vi "Mesh Page.vi"() -> ()   [LabVIEW 2017, in "3D Mesh.lvclass"]
uses:
  <vilib>/Math Plots/3D Math Plots/3D Mesh/3D Mesh/3D Mesh.lvclass
  <vilib>/Math Plots/3D Math Plots/3D Mesh/3D Mesh/Typedef/3D Mesh Propery Array.ctl
  <vilib>/Math Plots/3D Math Plots/3D Mesh/3D Mesh/Typedef/3D Mesh Property.ctl
  <vilib>/Math Plots/3D Math Plots/3D Plot/3D Plot/Typedef/Line Type.ctl
  <vilib>/Math Plots/3D Math Plots/3D Plot/3D Plot/Typedef/Color Ramp Cluster.ctl
  <vilib>/Math Plots/3D Math Plots/3D Plot/3D Plot/Typedef/Dialog State.ctl
  <vilib>/Math Plots/3D Math Plots/3D Plot/3D Plot/Typedef/Temp Scene State.ctl
  <vilib>/Math Plots/3D Math Plots/3D Plot/3D Plot/Typedef/Temp Scene Property Action.ctl
  <vilib>/Math Plots/3D Math Plots/3D Plot/3D Plot/3D Plot.lvclass
panel:
  in  "Mesh Mode":u16(ring)=2 caption="Mesh mode" items=["Lines", "Hidden Lines", "With Zero Plane"]
  in  "Line Style":u16(ring) caption="Line style"
  in  "Antialiasing":bool
  in  "Line Width":sgl=0.001 caption="Line width" min=0.001 step=1
  in  "Fill Color":u32(colorbox) caption="Fill color"
  out "Mesh Property Out":T1
  in  "Mesh Property In":T1
  out "Color Ramp":dbl[][](graph)
  in  "Color Map Style":u16(ring) caption="Color map style" items=["None ", "Shaded", "Color spectrum", "Grey scale", "Custom"]
  in  "YZ Plane Projection":bool caption="YZ plane projection"
  in  "XZ Plane Projection":bool caption="XZ plane projection"
  in  "XY Plane Projection":bool caption="XY plane projection"
  in  "Coordinate System":u16(ring) caption="Coordinate system" items=["Cartesian", "Cylindrical", "Spherical"]
  in  "Plot Opacity":sgl(slide) caption="Plot opacity(%)" min=0 max=100 scale=0.0..100.0
  in  "Plot List":i32(listbox)
  in  "Ramp Edit":bool caption="Ramp edit"
  in  "Move Down":bool
  in  "Move Up":bool
  in  "Delete":bool
  in  "New":bool
  in  "Event Registration":refnum<event-registration>
  # "Mesh"
  # "General"
  # "Projection"
  # "Color Ramp"
  # "Mesh"
  # "Surface"
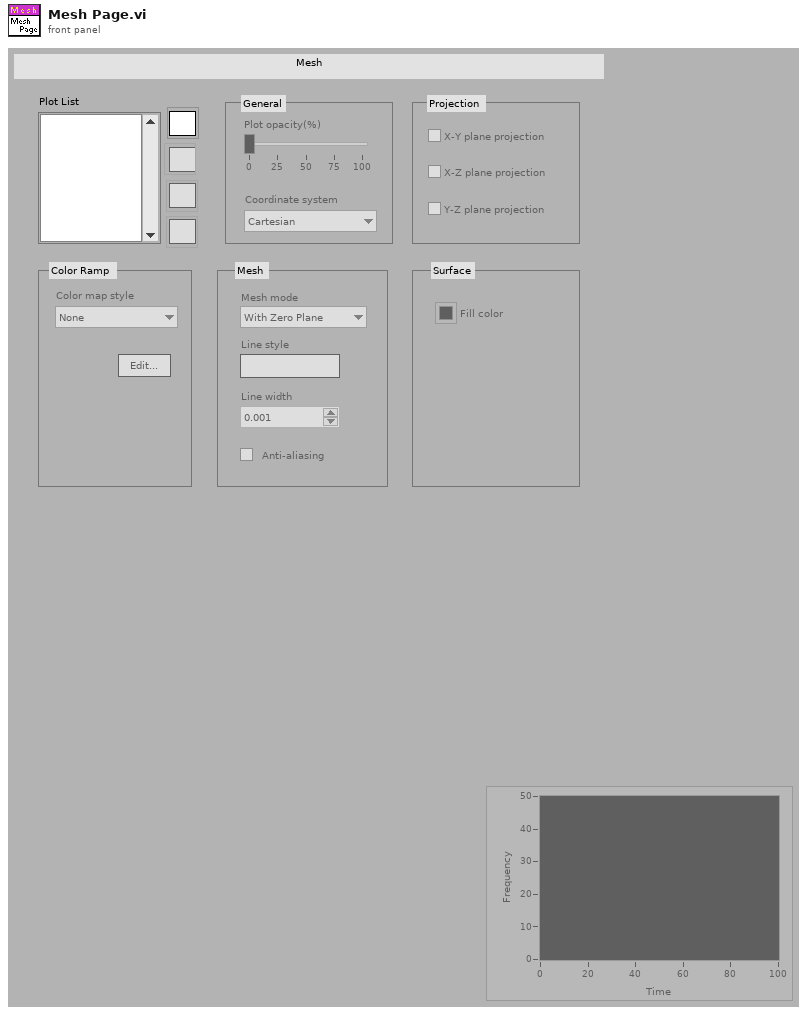
[diagram p1: front panel]
types:
  T1 = typedef "3D Mesh.lvclass/3D Mesh Propery Array.ctl" = T2[]
  T2 = typedef "3D Mesh.lvclass/3D Mesh Property.ctl" = cluster{"General Property":cluster{"Plot Name":string, "Coordinate System":enum16{"Cartesian", "Cylindrical", "Spherical"}, "Opacity":sgl}, "Projection Property":cluster{"Draw XY":bool, "Draw YZ":bool, "Draw XZ":bool}, "Plot Property":cluster{"Surface Color":u32, "Line Style":T3, "Line Width":sgl, "Color Ramp Cluster":T4, "Antialiasing":bool}, "Mesh Property":cluster{"Mesh Mode":enum16{"Lines", "Hidden Lines", "With Zero Plane"}}}
  T3 = typedef "3D Plot.lvclass/Line Type.ctl" = enum16{"None", "Solid", "Dash", "Dot", "Dash Dot"}
  T4 = typedef "3D Plot.lvclass/Color Ramp Cluster.ctl" = cluster{"Color Ramp Style":enum16{"None", "Shaded", "Color spectrum", "Grey scale", "Custom"}, "Color Ramp Array":u32[], "Color Ramp Index":i32[], "Interpolate?":bool, "Logarithm?":bool}
  T5 = typedef "3D Plot.lvclass/Dialog State.ctl" = enum16{"Initialize", "Read Porperty", "Write Property", "Idle", "Exit"}
  T6 = typedef "3D Plot.lvclass/Temp Scene State.ctl" = enum16{"Create", "Update Scene", "Get Plot Representation", "Destory"}
  T7 = typedef "3D Plot.lvclass/Temp Scene Property Action.ctl" = enum16{"Graph Property", "Light Property", "Axis Property", "Value Pair Property", "Format Property", "Cursor Property", "Plot Specific Property"}
  T8 = typedef "3D Plot.lvclass/Multiplot Representation.ctl" = cluster{"Plot Represention Array":T9[], "Max Range":T10}
  T9 = typedef "3D Plot.lvclass/Plot Representation.ctl" = cluster{"Plot ID":i32, "Plot Range":T10, "Mesh Data":T11, "Dimension":cluster{"X Dimension":i32, "Y Dimension":i32}, "Ramp Range":T10}
  T10 = typedef "3D Plot.lvclass/Range Clusters.ctl" = cluster{"X Range":cluster{"Max X":sgl, "Min X":sgl}, "Y Range":cluster{"Max Y":sgl, "Min Y":sgl}, "Z Range":cluster{"Max Z":sgl, "Min Z":sgl}}
  T11 = typedef "3D Plot.lvclass/Mesh Data.ctl" = cluster{"Index Array":u32[], "Vertex Array":cluster{"X":sgl, "Y":sgl, "Z":sgl}[], "Normal Array":cluster{"X":sgl, "Y":sgl, "Z":sgl}[], "Color Index Array":i32[]}
  T12 = enum16{"None", "Shaded", "Color spectrum", "Grey scale", "Custom"}
  T13 = enum16{"Lines", "Hidden Lines", "With Zero Plane"}
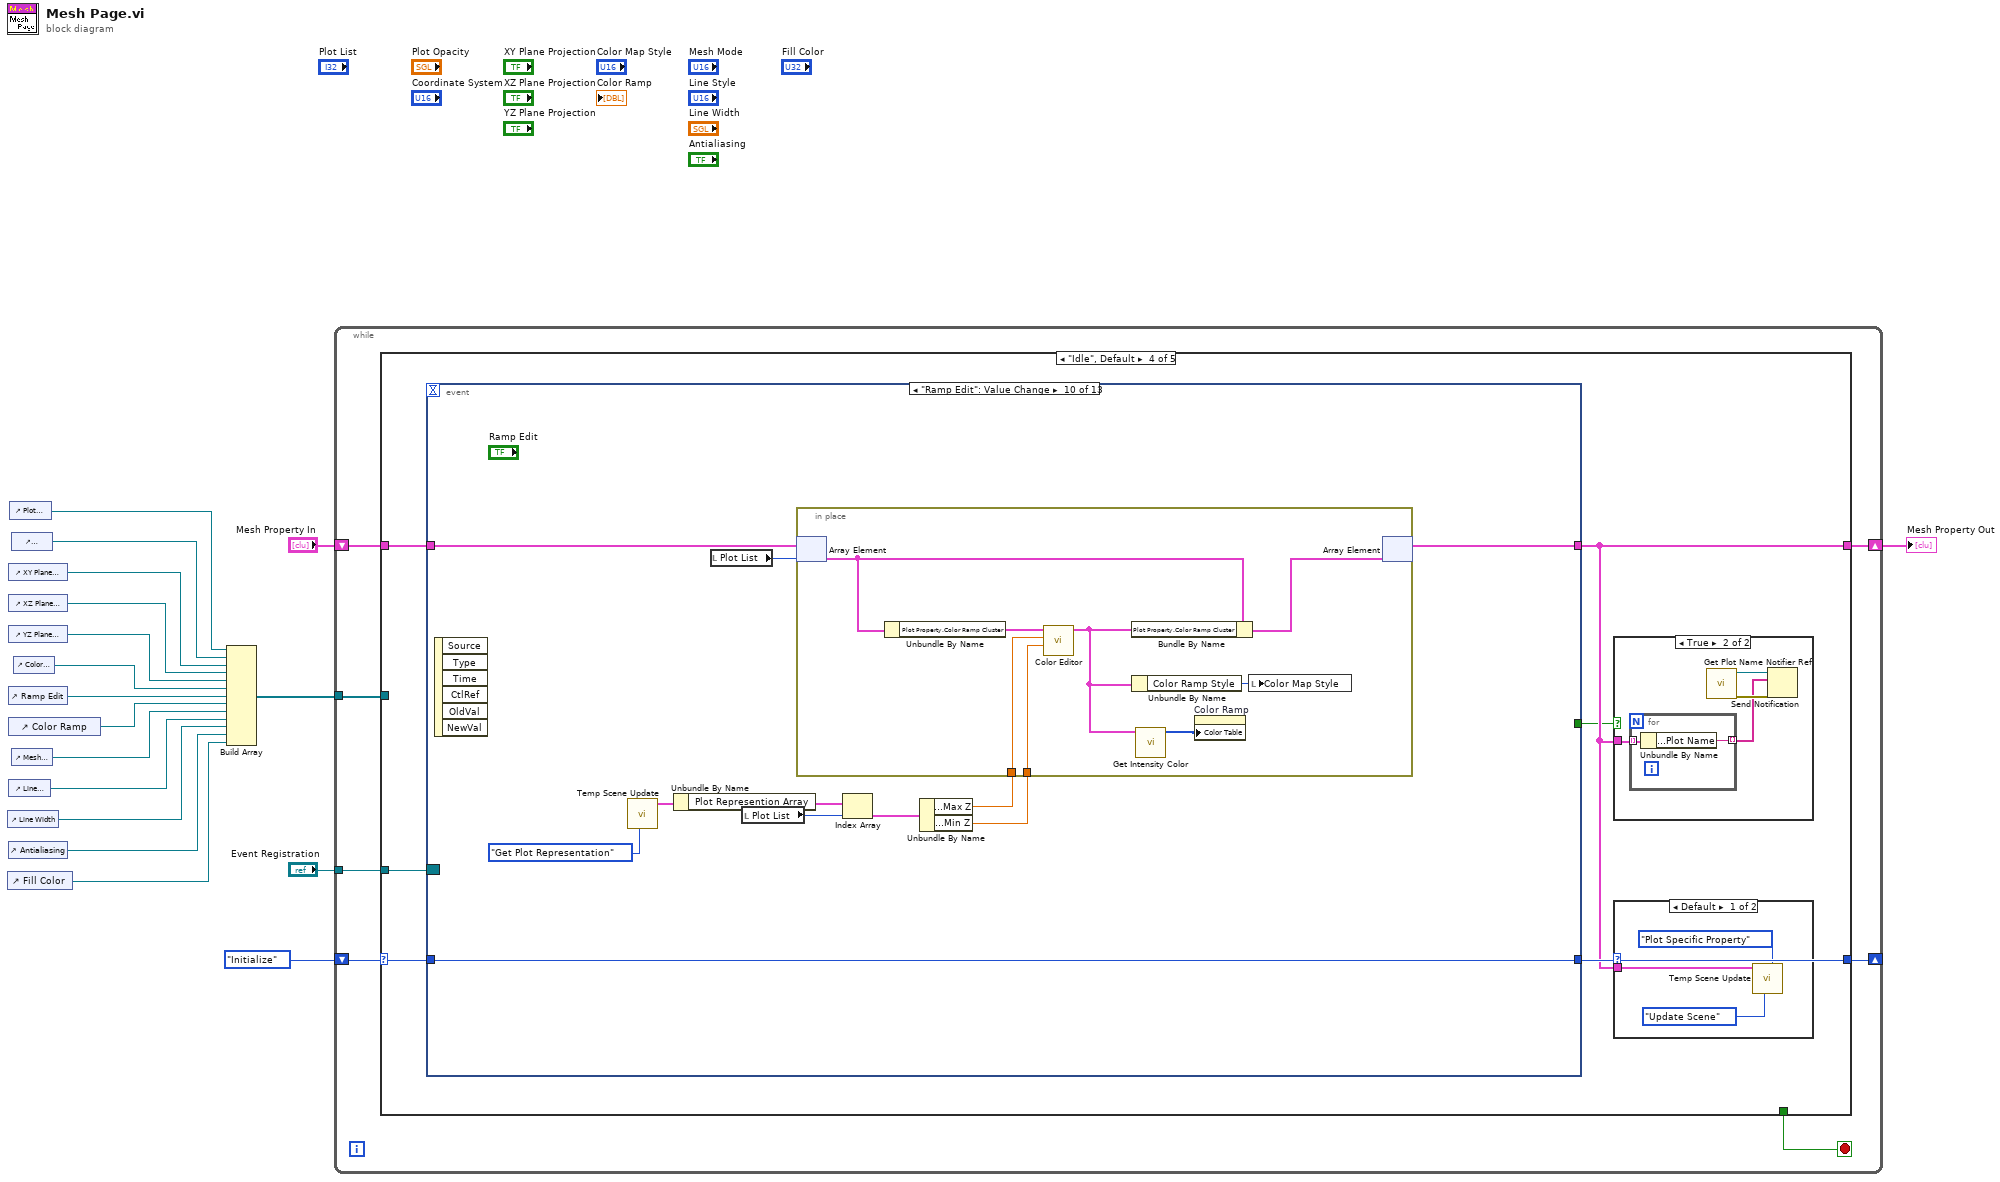
[diagram p0: block diagram]
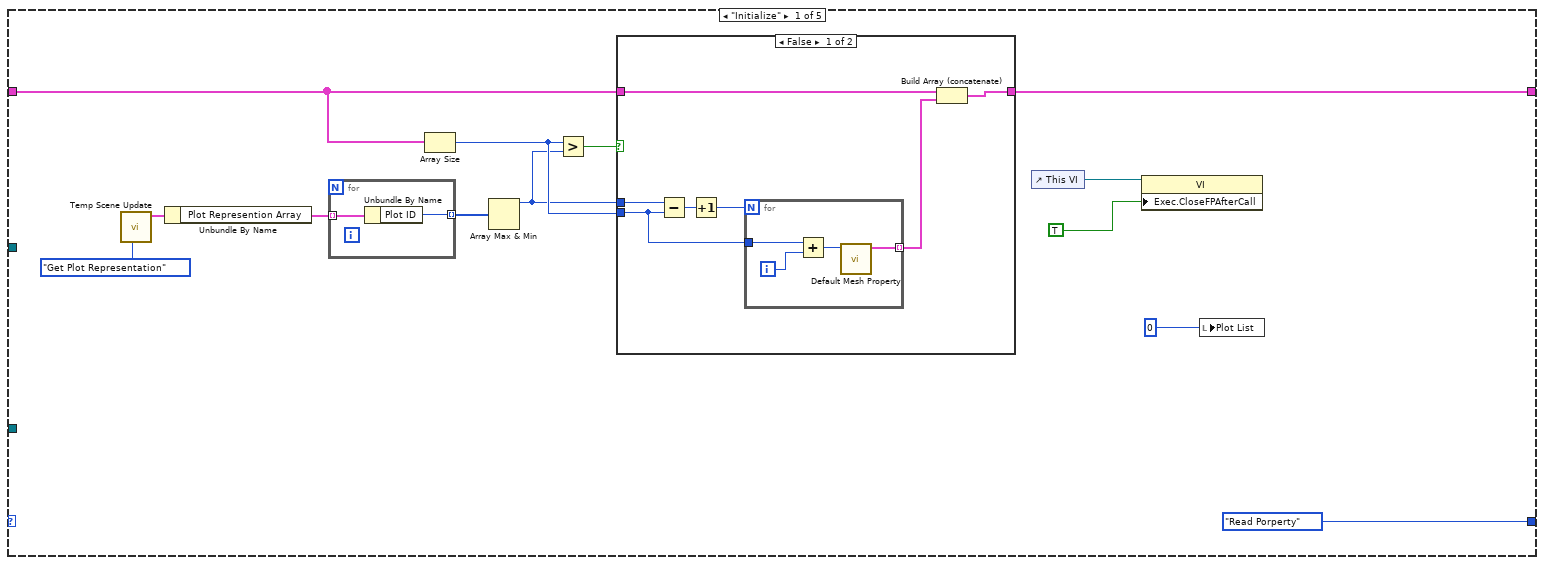
[diagram p2: hidden frame]
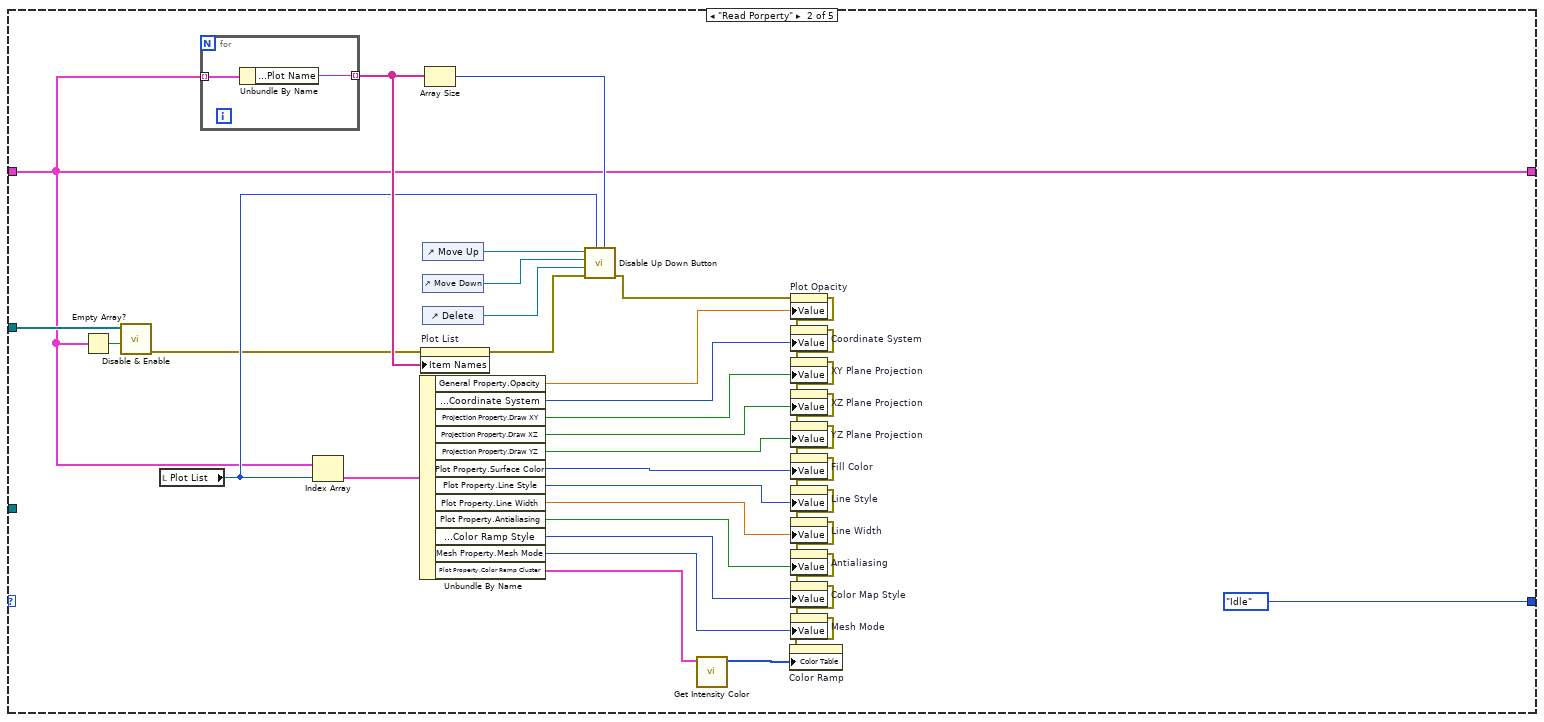
[diagram p4: hidden frame]
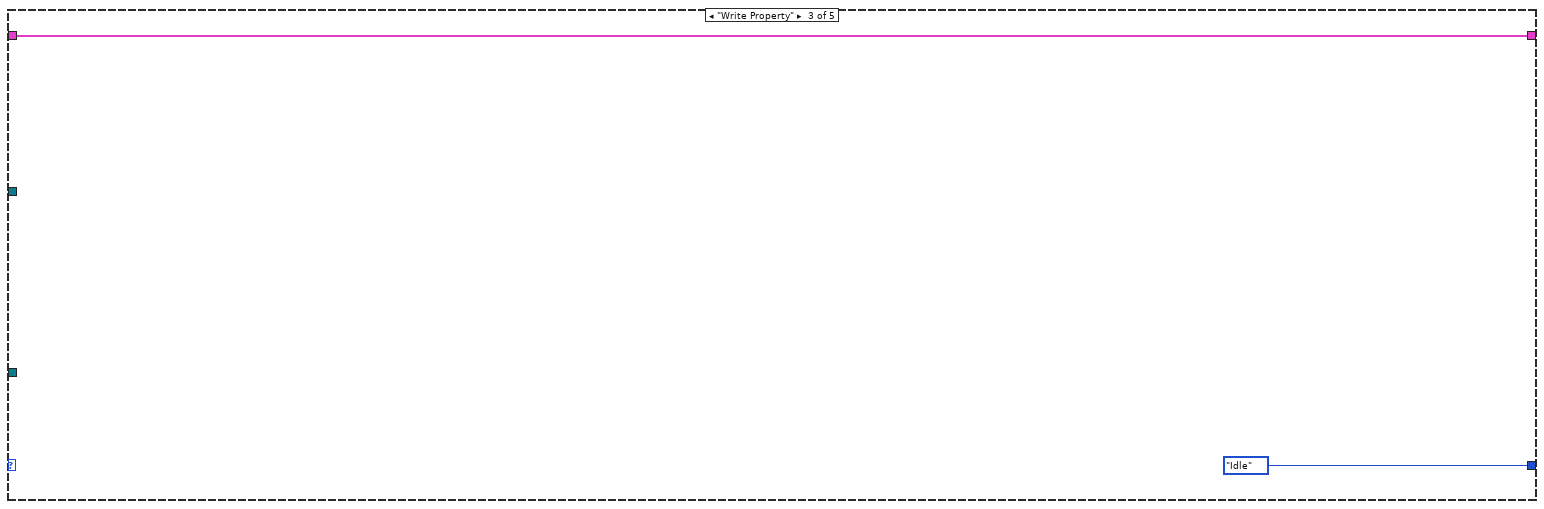
[diagram p5: hidden frame]
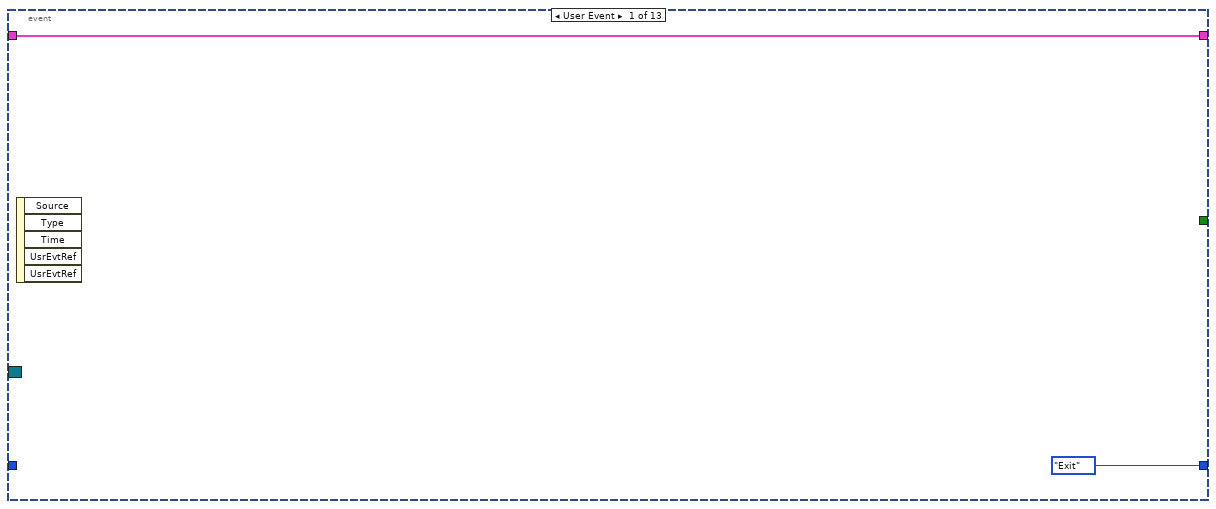
[diagram p8: hidden frame]
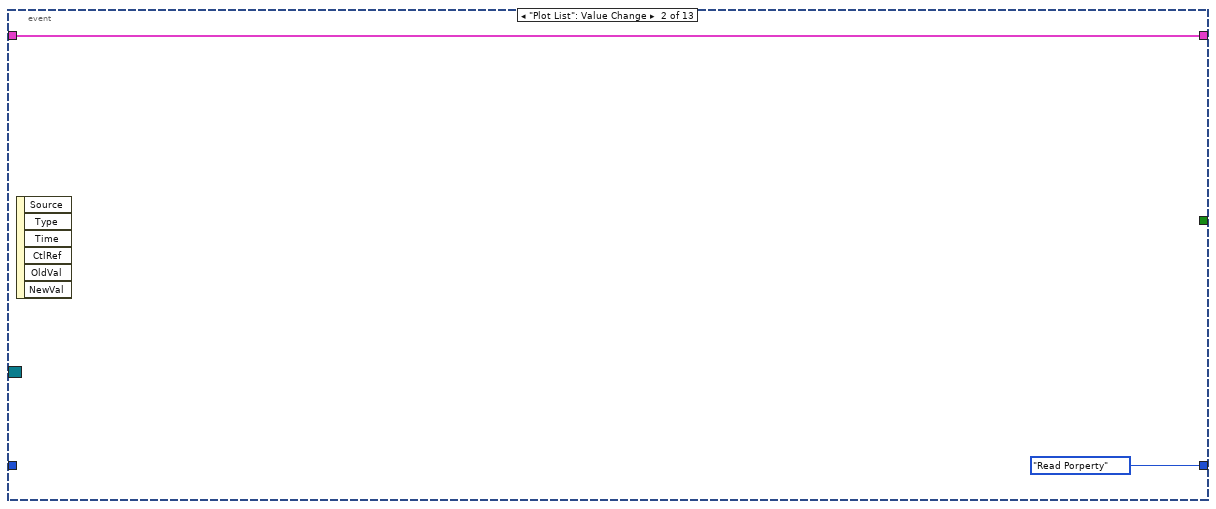
[diagram p9: hidden frame]
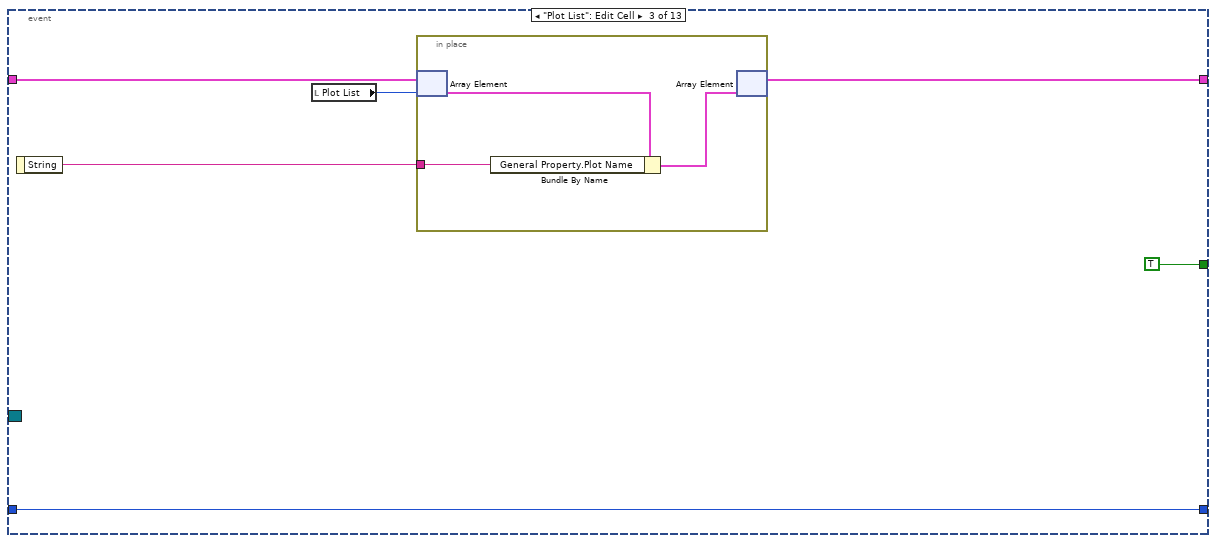
[diagram p10: hidden frame]
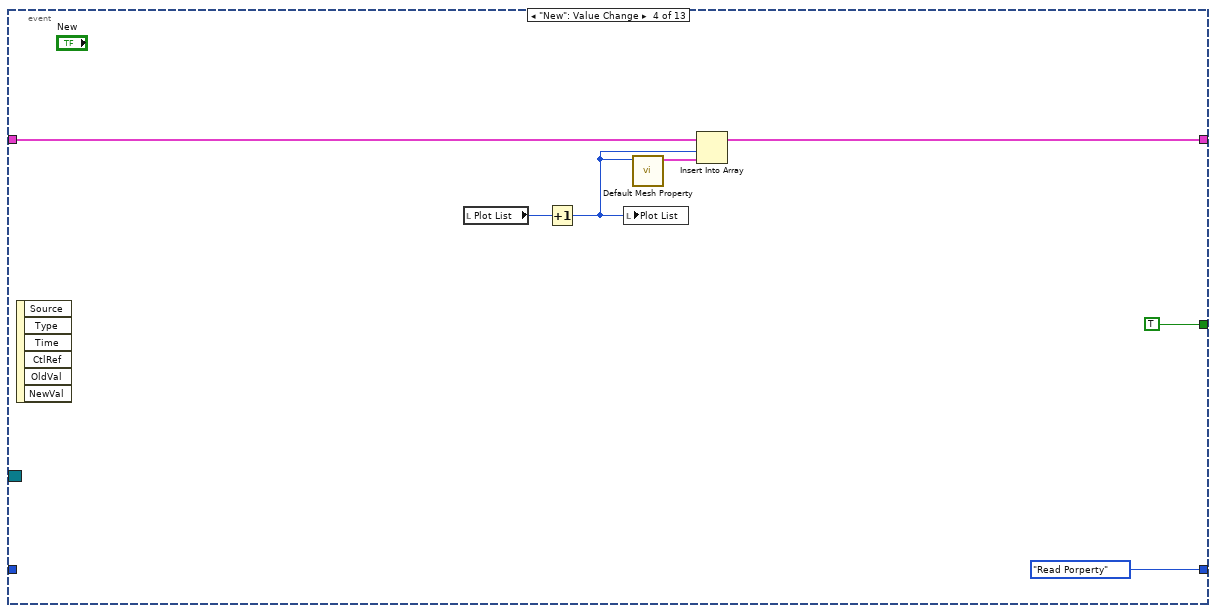
[diagram p11: hidden frame]
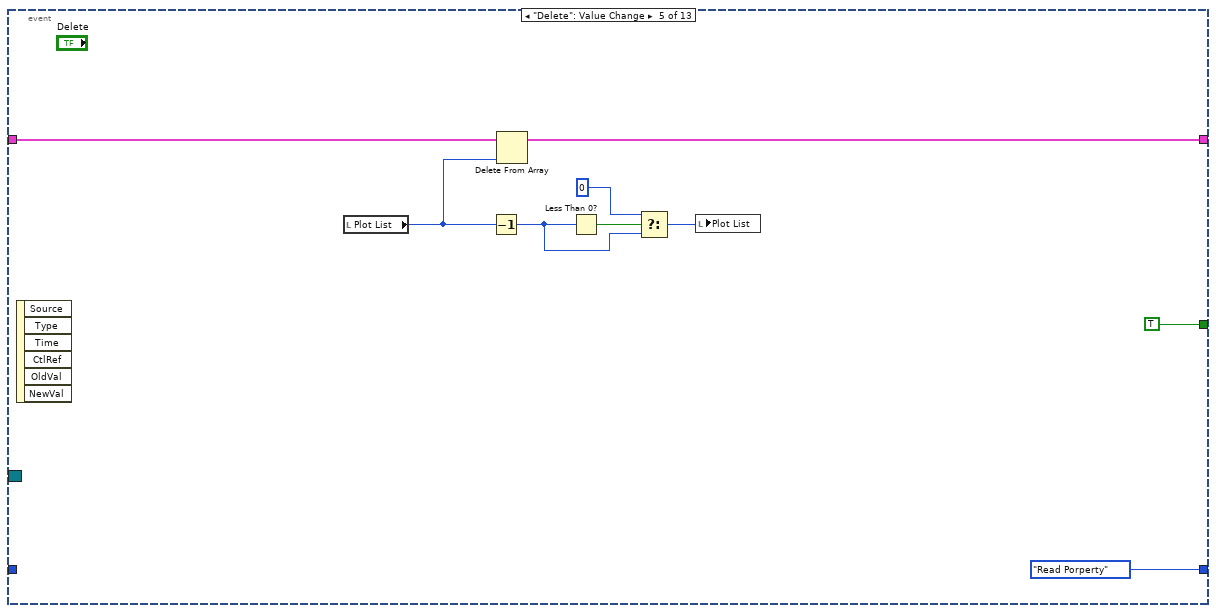
[diagram p12: hidden frame]
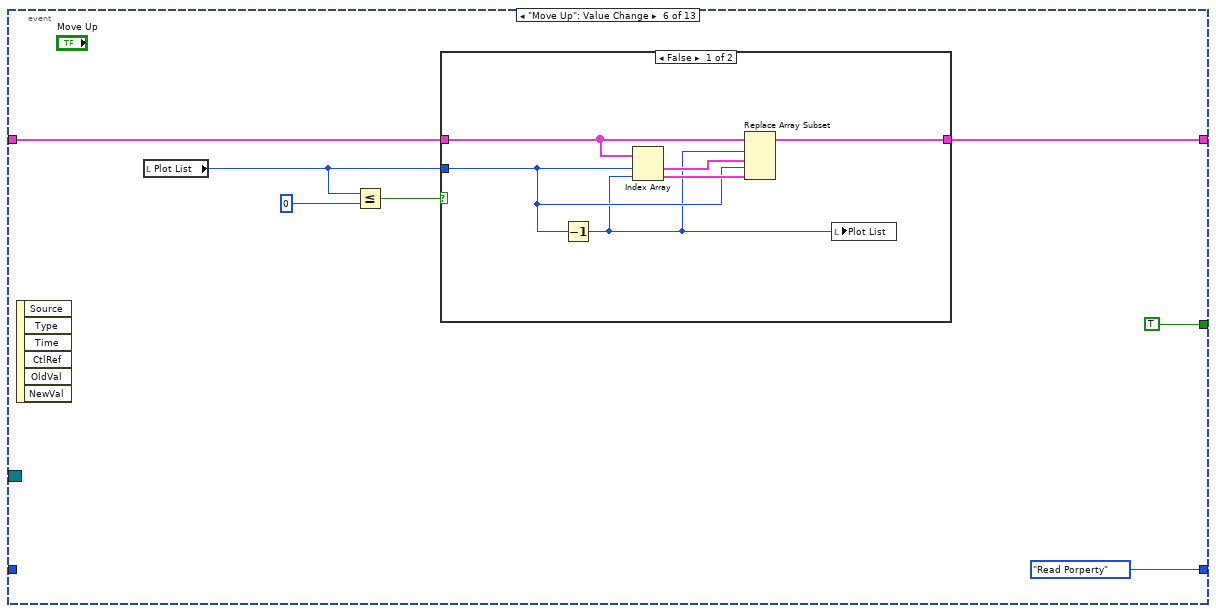
[diagram p13: hidden frame]
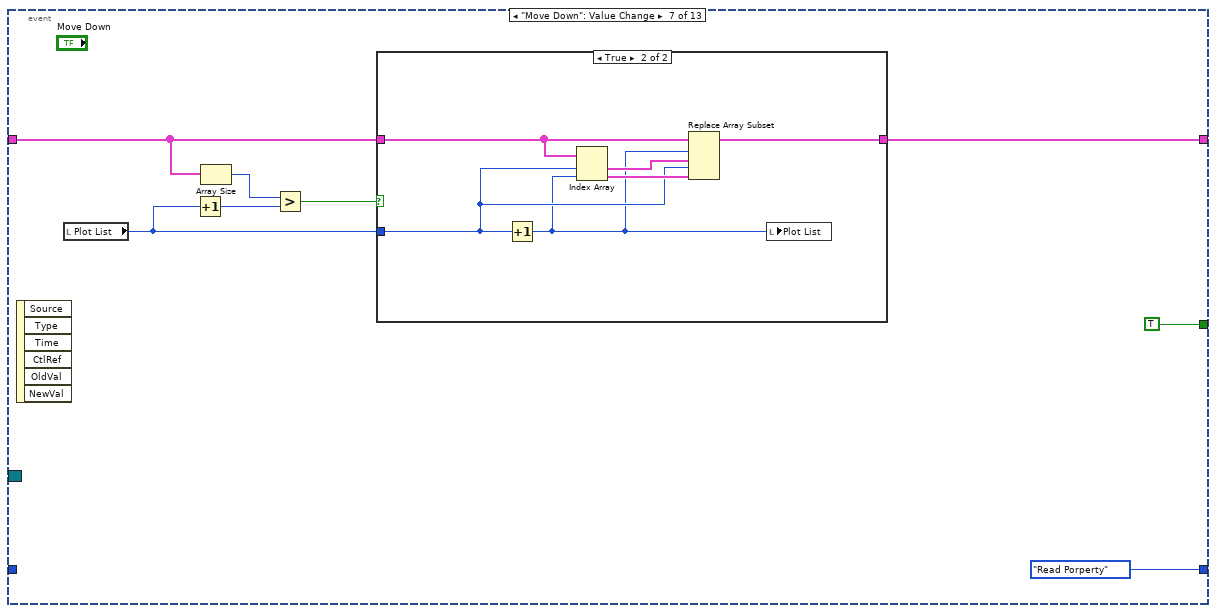
[diagram p15: hidden frame]
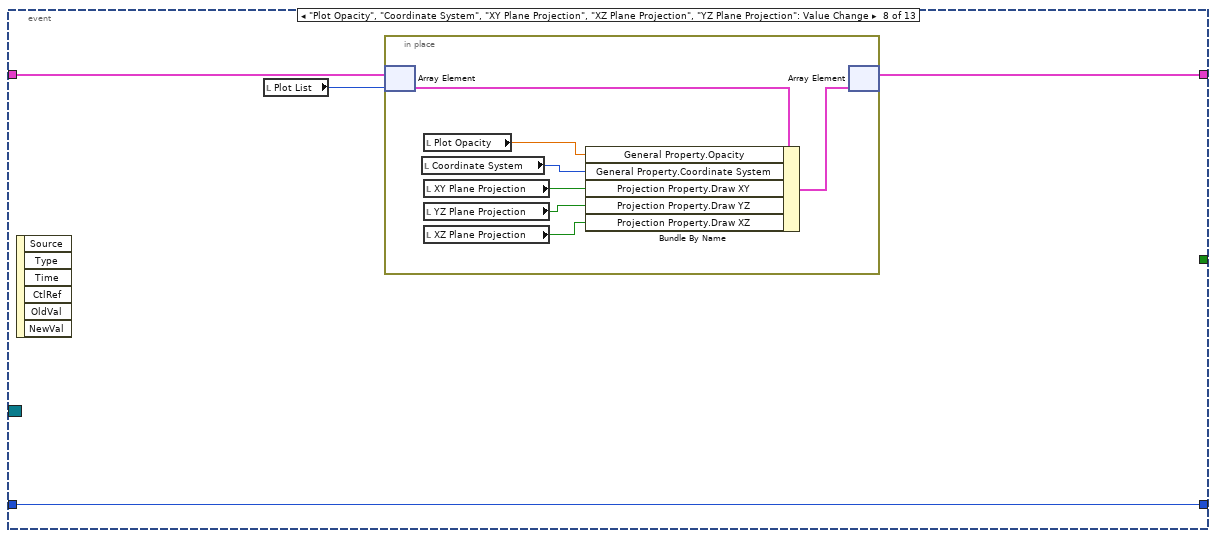
[diagram p17: hidden frame]
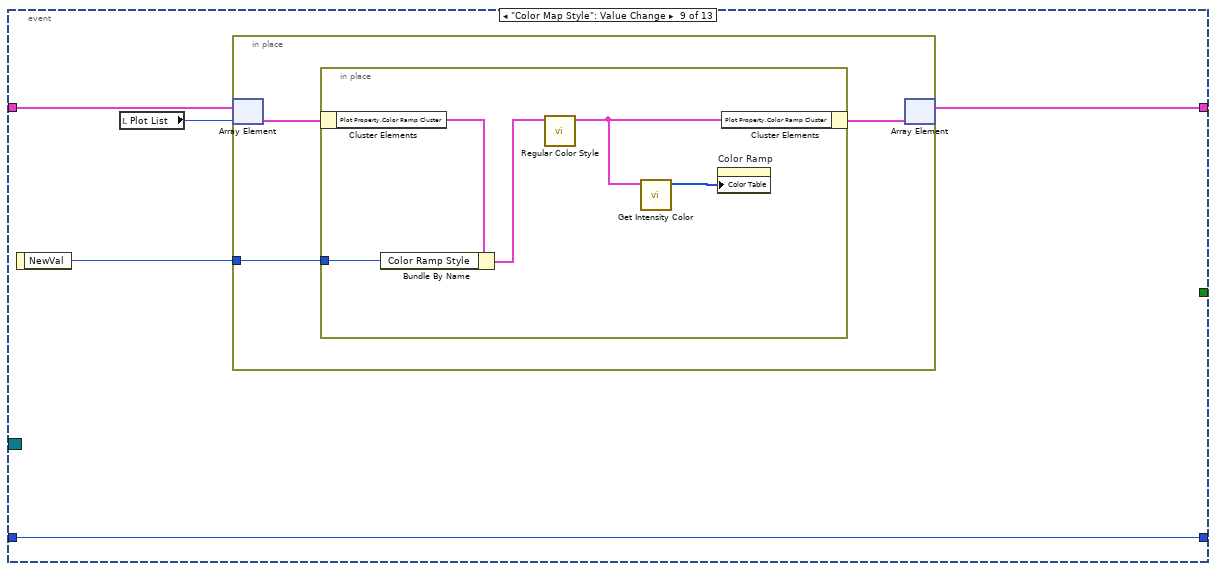
[diagram p18: hidden frame]
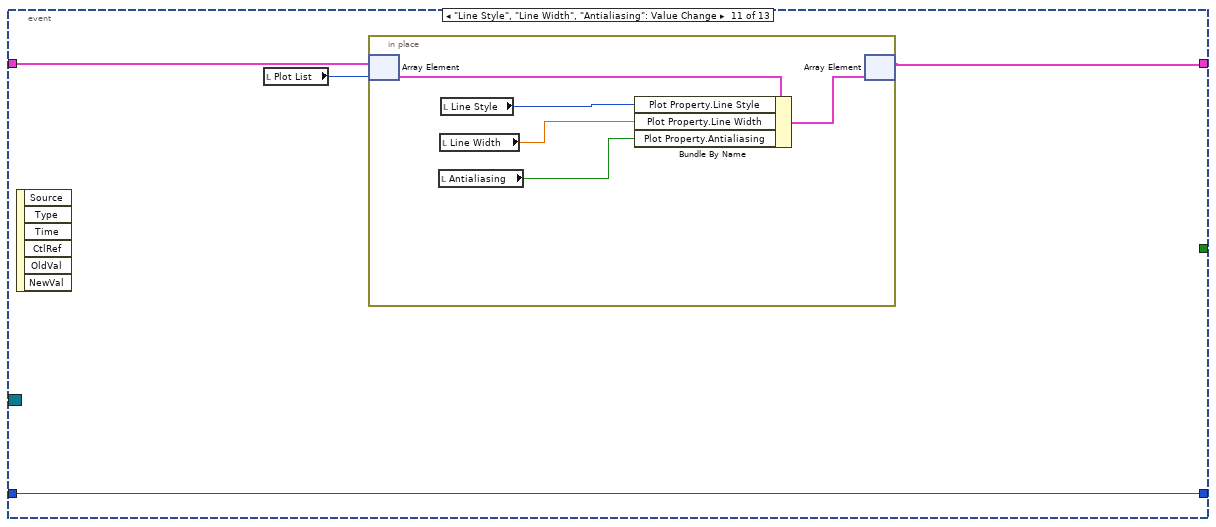
[diagram p19: hidden frame]
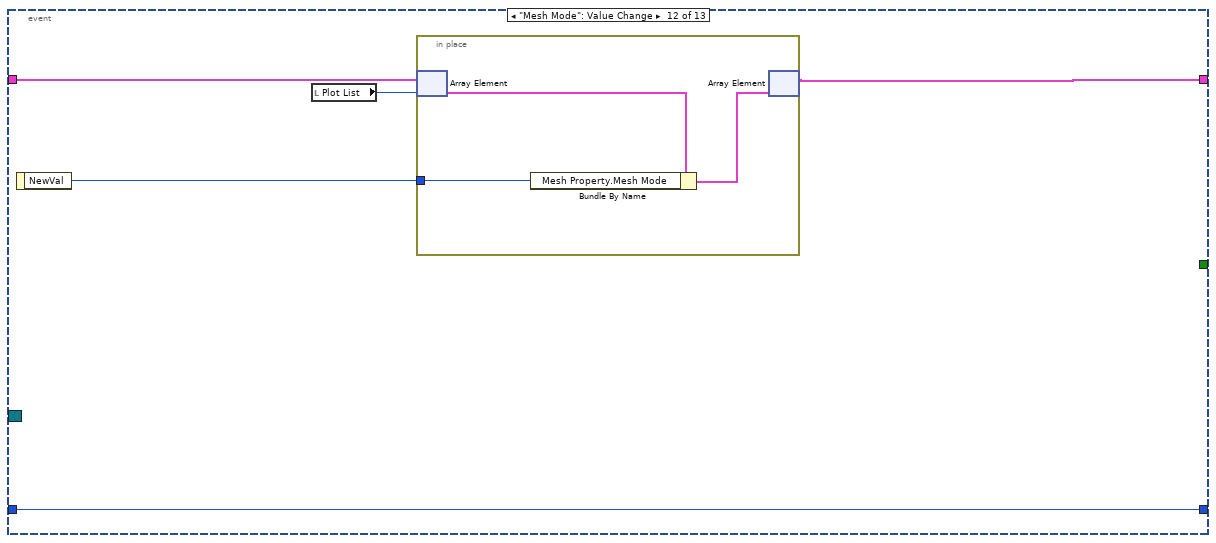
[diagram p20: hidden frame]
diagram:
  n1 = control-ref of="Line Width"() -> (w4:refnum<vi>)
  n2 = control-ref of="Fill Color"() -> (w2:refnum<vi>)
  n3 = control-ref of="XY Plane Projection"() -> (w12:refnum<vi>)
  n4 = control-ref of="XZ Plane Projection"() -> (w11:refnum<vi>)
  n5 = control-ref of="YZ Plane Projection"() -> (w10:refnum<vi>)
  n6 = control-ref of="Ramp Edit"() -> (w8:refnum<vi>)
  n7 = control-ref of="Color Ramp"() -> (w7:refnum<vi>)
  n8 = control-ref of="Line Style"() -> (w5:refnum<vi>)
  n9 = control-ref of="Antialiasing"() -> (w3:refnum<vi>)
  n10 = control-ref of="Plot Opacity"() -> (w14:refnum<vi>)
  n11 = control-ref of="Coordinate System"() -> (w13:refnum<vi>)
  n12 = control-ref of="Mesh Mode"() -> (w6:refnum<vi>)
  n13 = control-ref of="Color Map Style"() -> (w9:refnum<vi>)
  n14 = Build Array(w14, w13, w12, w11, w10, w9, w8, w7, w6, w5, w4, w3, w2) -> (w1:refnum<vi>[])
  n15 = while {
    shift-right: [w24] -> w15
    shift-left: "Mesh Property In" -> [w25]
    shift-right: [w20] -> _
    shift-left: Dialog_State."Initialize" -> [w23]
    tunnel: "Event Registration" -> [w21]
    tunnel: w1 -> [w19]
    stop <- w22 stop-if-true
    n16 = case shown="\"Idle\", Default" w23 {
      selector: w23 -> [_ _ _ w98 _]
      tunnel: w25 -> [w28 w77 w93 w100 w236]
      tunnel: [w27 w77 w93 w96 w236] -> w24
      tunnel: [Dialog_State."Read Porperty" Dialog_State."Idle" Dialog_State."Idle" w97 Dialog_State."Exit"] -> w20
      tunnel: [_ _ _ _ TRUE] -> w22
      tunnel: w21 -> [_ _ _ w99 _]
      tunnel: w19 -> [_ w79 _ _ _]
      frame "Initialize" {
        n17 = call <vilib>:"Temp Scene Update.vi"("State"=Temp_Scene_State."Get Plot Representation") -> ("Multiplot Representation"=w33:T8)  [unwired: 5 in, 5 out]
        n18 = Unbundle By Name(w33) -> ("Plot Represention Array"=w26:T9[])
        n19 = for {
          tunnel: w26 -> [w52] mode=indexing
          tunnel: [w51] -> w32 mode=indexing
          n20 = Unbundle By Name(w52) -> ("Plot ID"=w51:i32)
        }
        n21 = Array Size(array=w28) -> (size(s)=w30:i32)
        n22 = Array Max & Min(array=w32) -> (max value=w29:i32)  [unwired: 3 out]
        n23 = Greater?(x=w30, y=w29) -> (0:w31:bool)
        n24 = case shown="False" w31 {
          tunnel: [w43 w50] -> w27
          tunnel: w28 -> [w45 w50]
          tunnel: w30 -> [w39 _]
          tunnel: w29 -> [w40 _]
          frame False {
            n25 = Subtract(x=w40, y=w39) -> (x-y=w42:i32)
            n26 = Increment(x=w42) -> (x+1=w41:i32)
            n27 = for {
              N: w41 -> [_]
              tunnel: w39 -> [w48]
              tunnel: [w46] -> w44 mode=indexing
              i -> [w49]
              n28 = Add(x=w48, y=w49) -> (x+y=w47:i32)
              n29 = call <vilib>:"Default Mesh Property.vi"("Plot ID"=w47) -> ("Default Property"=w46:T2)  [unwired: 10 out]
            }
            n30 = Build Array (concatenate)(w45, w44) -> (w43:T1)
          }
          frame True {
          }
        }
        n31 = control-ref of="This VI"() -> (w37:refnum<vi>)
        n32 = property class="VI"(reference=w37, "Exec.CloseFPAfterCall"=TRUE ("Execution:Close After Call")) -> ()  [unwired: 1 in, 2 out]
        n33 = local write "Plot List"(0 ("Plot List")) -> ()
      }
      frame "Read Porperty" {
        n34 = Empty Array?(array=w77) -> (empty?=w78:bool)
        n35 = call <vilib>:"Disable & Enable.vi"("Disabled?"=w78, "Control Ref Array"=w79) -> ("error out"=w76:errorcluster)  [unwired: 1 in, 8 out]
        n36 = local read "Plot List"() -> (w80:i32)
        n37 = for {
          tunnel: w77 -> [w92] mode=indexing
          tunnel: [w91] -> w82 mode=indexing
          n38 = Unbundle By Name(w92) -> ("General Property.Plot Name"=w91:string)
        }
        n39 = Index Array(array=w77, index=w80) -> (element=w89:T2)
        n40 = Unbundle By Name(w89) -> ("General Property.Opacity"=w65:sgl, "General Property.Coordinate System"=w64:enum16{"Cartesian", "Cylindrical", "Spherical"}, "Projection Property.Draw XY"=w63:bool, "Projection Property.Draw XZ"=w62:bool, "Projection Property.Draw YZ"=w61:bool, "Plot Property.Surface Color"=w60:u32, "Plot Property.Line Style"=w59:T3, "Plot Property.Line Width"=w58:sgl, "Plot Property.Antialiasing"=w57:bool, "Plot Property.Color Ramp Cluster.Color Ramp Style"=w56:T12, "Mesh Property.Mesh Mode"=w55:T13, "Plot Property.Color Ramp Cluster"=w88:T4)
        n41 = property on="Plot List" class="LstBox (strict)"(error in=w76, "Item Names"=w82) -> (error out=w81:errorcluster)  [unwired: 1 in, 1 out]
        n42 = control-ref of="Move Up"() -> (w84:refnum<vi>)
        n43 = control-ref of="Move Down"() -> (w85:refnum<vi>)
        n44 = control-ref of="Delete"() -> (w86:refnum<vi>)
        n45 = Array Size(array=w82) -> (size(s)=w83:i32)
        n46 = call <vilib>:"Disable Up Down Button.vi"("Length"=w83, "Index"=w80, "error in (no error)"=w81, "Delete Ref"=w86, "Move Down Ref"=w85, "Move Up Ref"=w84) -> ("error out"=w53:errorcluster)  [unwired: 5 out]
        n47 = call <vilib>:"Get Intensity Color.vi"("Color Ramp Cluster"=w88) -> ("Intensity Color"=w87:u32[])  [unwired: 4 in, 6 out]
        n48 = property on="Plot Opacity" class="Slide (strict)"(error in=w53, "Value"=w65) -> (error out=w75:errorcluster)  [unwired: 1 in, 1 out]
        n49 = property on="Coordinate System" class="Ring (strict)"(error in=w75, "Value"=w64) -> (error out=w74:errorcluster)  [unwired: 1 in, 1 out]
        n50 = property on="XY Plane Projection" class="Bool (strict)"(error in=w74, "Value"=w63) -> (error out=w73:errorcluster)  [unwired: 1 in, 1 out]
        n51 = property on="XZ Plane Projection" class="Bool (strict)"(error in=w73, "Value"=w62) -> (error out=w72:errorcluster)  [unwired: 1 in, 1 out]
        n52 = property on="YZ Plane Projection" class="Bool (strict)"(error in=w72, "Value"=w61) -> (error out=w71:errorcluster)  [unwired: 1 in, 1 out]
        n53 = property on="Fill Color" class="ColBox"(error in=w71, "Value"=w60) -> (error out=w70:errorcluster)  [unwired: 1 in, 1 out]
        n54 = property on="Line Style" class="Ring (strict)"(error in=w70, "Value"=w59) -> (error out=w69:errorcluster)  [unwired: 1 in, 1 out]
        n55 = property on="Line Width" class="DigNum (strict)"(error in=w69, "Value"=w58) -> (error out=w68:errorcluster)  [unwired: 1 in, 1 out]
        n56 = property on="Antialiasing" class="Bool (strict)"(error in=w68, "Value"=w57) -> (error out=w67:errorcluster)  [unwired: 1 in, 1 out]
        n57 = property on="Color Map Style" class="Ring (strict)"(error in=w67, "Value"=w56) -> (error out=w66:errorcluster)  [unwired: 1 in, 1 out]
        n58 = property on="Mesh Mode" class="Ring (strict)"(error in=w66, "Value"=w55) -> (error out=w54:errorcluster)  [unwired: 1 in, 1 out]
        n59 = property on="Color Ramp" class="IntGraph (strict)"(error in=w54, "Color Table"=w87) -> ()  [unwired: 1 in, 2 out]
      }
      frame "Write Property" {
      }
      frame "Idle", Default {
        n60 = event shown="[9] \"Ramp Edit\": Value Change" {
          selector: w99 -> [_ _ _ _ _ _ _ _ _ _ _ _ _]
          dyn-events: _ -> [_ _ _ _ _ _ _ _ _ _ _ _ _]
          timeout: _ -> [_ _ _ _ _ _ _ _ _ _ _ _ _]
          tunnel: w100 -> [w111 w113 w117 w127 w136 w141 w155 w169 w182 w200 w212 w222 w230]
          tunnel: [w111 w113 w116 w126 w137 w140 w154 w168 w181 w199 w211 w221 w229] -> w96
          tunnel: [Dialog_State."Exit" Dialog_State."Read Porperty" w115 Dialog_State."Read Porperty" Dialog_State."Read Porperty" Dialog_State."Read Porperty" Dialog_State."Read Porperty" w171 w183 w202 w214 w223 w231] -> w97
          tunnel: w98 -> [_ _ w115 _ _ _ _ w171 w183 w202 w214 w223 w231]
          tunnel: [_ _ TRUE TRUE TRUE TRUE TRUE _ _ _ _ _ _] -> w95
          event User Event {
            n61 = event-data() -> ()  [unwired: 6 out]
          }
          event "Plot List": Value Change {
            n62 = event-data() -> ()  [unwired: 7 out]
          }
          event "Plot List": Edit Cell {
            n63 = event-data() -> ("String"=w118:string)  [unwired: 1 out]
            n64 = local read "Plot List"() -> (w119:i32)
            n65 = in-place {
              in-place-border: w118 -> [w120]
              n66 = in-place-array #1(w117, w119) -> (w122:T2)
              n67 = Bundle By Name(cluster=w122, "General Property.Plot Name"=w120) -> (w121:T2)
              n68 = in-place-array #1(w121) -> (w116:T1)  [unwired: 1 out]
            }
          }
          event "New": Value Change {
            n69 = event-data() -> ()  [unwired: 7 out]
            n70 = local read "Plot List"() -> (w128:i32)
            n71 = Increment(x=w128) -> (x+1=w124:i32)
            n72 = local write "Plot List"(w124) -> ()
            n73 = call <vilib>:"Default Mesh Property.vi"("Plot ID"=w124) -> ("Default Property"=w123:T2)  [unwired: 10 out]
            n74 = Insert Into Array(array=w127, index=w124, new element=w123) -> (w126:T1)
          }
          event "Delete": Value Change {
            n75 = event-data() -> ()  [unwired: 7 out]
            n76 = local read "Plot List"() -> (w132:i32)
            n77 = Decrement(x=w132) -> (x-1=w133:i32)
            n78 = Delete From Array(array=w136, index=w132) -> (array with subset deleted=w137:T1)  [unwired: 1 in, 1 out]
            n79 = Less Than 0?(x=w133) -> (x < 0?=w135:bool)
            n80 = Select(t=0, s=w135, f=w133) -> (s? t:f=w131:i32)
            n81 = local write "Plot List"(w131) -> ()
          }
          event "Move Up": Value Change {
            n82 = event-data() -> ()  [unwired: 7 out]
            n83 = local read "Plot List"() -> (w142:i32)
            n84 = Less Or Equal?(x=w142, y=0) -> (x <= y?=w144:bool)
            n85 = case shown="False" w144 {
              tunnel: w141 -> [w149 w152]
              tunnel: [w148 w152] -> w140
              tunnel: w142 -> [w147 _]
              frame False {
                n86 = Decrement(x=w147) -> (x-1=w146:i32)
                n87 = Index Array(array=w149, index #1=w147, index #2=w146) -> (element #1=w151:T2, element #2=w150:T2)
                n88 = Replace Array Subset(array=w149, new element #1=w151, index #1=w146, new element #2=w150, index #2=w147) -> (w148:T1)
                n89 = local write "Plot List"(w146) -> ()
              }
              frame True {
                # "List value is less or equal to 0.\nThe active item is in the top of the list."
              }
            }
          }
          event "Move Down": Value Change {
            n90 = event-data() -> ()  [unwired: 7 out]
            n91 = local read "Plot List"() -> (w156:i32)
            n92 = Increment(x=w156) -> (x+1=w158:i32)
            n93 = Array Size(array=w155) -> (size(s)=w157:i32)
            n94 = Greater?(x=w157, y=w158) -> (0:w159:bool)
            n95 = case shown="True" w159 {
              tunnel: w155 -> [w161 w165]
              tunnel: [w161 w164] -> w154
              tunnel: w156 -> [_ w163]
              frame False {
                # "List value +1 is not less array length.\nThe active item is in the buttom of the list."
              }
              frame True {
                n96 = Increment(x=w163) -> (x+1=w162:i32)
                n97 = Index Array(array=w165, index #1=w163, index #2=w162) -> (element #1=w167:T2, element #2=w166:T2)
                n98 = Replace Array Subset(array=w165, new element #1=w167, index #1=w162, new element #2=w166, index #2=w163) -> (w164:T1)
                n99 = local write "Plot List"(w162) -> ()
              }
            }
          }
          event "Plot Opacity", "Coordinate System", "XY Plane Projection", "XZ Plane Projection", "YZ Plane Projection": Value Change {
            n100 = event-data() -> ()  [unwired: 7 out]
            n101 = local read "Plot List"() -> (w170:i32)
            n102 = in-place {
              n103 = in-place-array #2(w169, w170) -> (w174:T2)
              n104 = local read "Coordinate System"() -> (w172:u16)
              n105 = local read "Plot Opacity"() -> (w178:sgl)
              n106 = local read "XY Plane Projection"() -> (w177:bool)
              n107 = local read "YZ Plane Projection"() -> (w175:bool)
              n108 = local read "XZ Plane Projection"() -> (w176:bool)
              n109 = Bundle By Name(cluster=w174, "General Property.Opacity"=w178, "General Property.Coordinate System"=w172, "Projection Property.Draw XY"=w177, "Projection Property.Draw YZ"=w175, "Projection Property.Draw XZ"=w176) -> (w173:T2)
              n110 = in-place-array #2(w173) -> (w168:T1)  [unwired: 1 out]
            }
          }
          event "Color Map Style": Value Change {
            n111 = event-data() -> ("NewVal"=w179:u16)  [unwired: 1 out]
            n112 = local read "Plot List"() -> (w180:i32)
            n113 = in-place {
              in-place-border: w179 -> [w185]
              n114 = in-place-array #3(w182, w180) -> (w186:T2)
              n115 = in-place {
                in-place-border: w185 -> [w190]
                n116 = in-place-cluster #4(w186) -> ("Plot Property.Color Ramp Cluster"=w191:T4)
                n117 = Bundle By Name(cluster=w191, "Color Ramp Style"=w190) -> (w189:T4)
                n118 = call <vilib>:"Regular Color Style.vi"("Color Ramp Cluster in"=w189) -> ("Color Ramp Cluster out"=w187:T4)  [unwired: 10 in]
                n119 = call <vilib>:"Get Intensity Color.vi"("Color Ramp Cluster"=w187) -> ("Intensity Color"=w188:u32[])  [unwired: 4 in, 6 out]
                n120 = property on="Color Ramp" class="IntGraph (strict)"("Color Table"=w188) -> ()  [unwired: 2 in, 2 out]
                n121 = in-place-cluster #4("Plot Property.Color Ramp Cluster"=w187) -> (w184:T2)
              }
              n122 = in-place-array #3(w184) -> (w181:T1)  [unwired: 1 out]
            }
          }
          event "Ramp Edit": Value Change {
            n123 = event-data() -> ()  [unwired: 7 out]
            n124 = call <vilib>:"Temp Scene Update.vi"("State"=Temp_Scene_State."Get Plot Representation") -> ("Multiplot Representation"=w195:T8)  [unwired: 5 in, 5 out]
            n125 = Unbundle By Name(w195) -> ("Plot Represention Array"=w192:T9[])
            n126 = local read "Plot List"() -> (w201:i32)
            n127 = local read "Plot List"() -> (w198:i32)
            n128 = Index Array(array=w192, index=w198) -> (element=w197:T9)
            n129 = Unbundle By Name(w197) -> ("Plot Range.Z Range.Max Z"=w194:sgl, "Plot Range.Z Range.Min Z"=w193:sgl)
            n130 = in-place {
              in-place-border: w194 -> [w206]
              in-place-border: w193 -> [w205]
              n131 = in-place-array #5(w200, w201) -> (w209:T2)
              n132 = Unbundle By Name(w209) -> ("Plot Property.Color Ramp Cluster"=w208:T4)
              n133 = call <vilib>:"Color Editor.vi"("Min"=w205, "Max"=w206, "Color Ramp Cluster in"=w208) -> ("Color Ramp Cluster out"=w204:T4)  [unwired: 3 in, 5 out]
              n134 = Bundle By Name(cluster=w209, "Plot Property.Color Ramp Cluster"=w204) -> (w210:T2)
              n135 = Unbundle By Name(w204) -> ("Color Ramp Style"=w203:T12)
              n136 = call <vilib>:"Get Intensity Color.vi"("Color Ramp Cluster"=w204) -> ("Intensity Color"=w207:u32[])  [unwired: 4 in, 6 out]
              n137 = property on="Color Ramp" class="IntGraph (strict)"("Color Table"=w207) -> ()  [unwired: 2 in, 2 out]
              n138 = local write "Color Map Style"(w203) -> ()
              n139 = in-place-array #5(w210) -> (w199:T1)  [unwired: 1 out]
            }
          }
          event "Line Style", "Line Width", "Antialiasing": Value Change {
            n140 = event-data() -> ()  [unwired: 7 out]
            n141 = local read "Plot List"() -> (w213:i32)
            n142 = in-place {
              n143 = in-place-array #6(w212, w213) -> (w216:T2)
              n144 = local read "Antialiasing"() -> (w217:bool)
              n145 = local read "Line Width"() -> (w218:sgl)
              n146 = local read "Line Style"() -> (w219:u16)
              n147 = Bundle By Name(cluster=w216, "Plot Property.Line Style"=w219, "Plot Property.Line Width"=w218, "Plot Property.Antialiasing"=w217) -> (w215:T2)
              n148 = in-place-array #6(w215) -> (w211:T1)  [unwired: 1 out]
            }
          }
          event "Mesh Mode": Value Change {
            n149 = event-data() -> ("NewVal"=w220:u16)  [unwired: 1 out]
            n150 = local read "Plot List"() -> (w224:i32)
            n151 = in-place {
              in-place-border: w220 -> [w225]
              n152 = in-place-array #7(w222, w224) -> (w227:T2)
              n153 = Bundle By Name(cluster=w227, "Mesh Property.Mesh Mode"=w225) -> (w226:T2)
              n154 = in-place-array #7(w226) -> (w221:T1)  [unwired: 1 out]
            }
          }
          event "Fill Color": Value Change {
            n155 = event-data() -> ("NewVal"=w228:u32)  [unwired: 1 out]
            n156 = local read "Plot List"() -> (w232:i32)
            n157 = in-place {
              in-place-border: w228 -> [w233]
              n158 = in-place-array #8(w230, w232) -> (w235:T2)
              n159 = Bundle By Name(cluster=w235, "Plot Property.Surface Color"=w233) -> (w234:T2)
              n160 = in-place-array #8(w234) -> (w229:T1)  [unwired: 1 out]
            }
          }
        }
        n161 = case shown="True" w95 {
          tunnel: w96 -> [_ w101]
          frame False {
          }
          frame True {
            n162 = for {
              tunnel: w101 -> [w106] mode=indexing
              tunnel: [w105] -> w102 mode=indexing
              n163 = Unbundle By Name(w106) -> ("General Property.Plot Name"=w105:string)
            }
            n164 = call <vilib>:"Get Plot Name Notifier Ref.vi"() -> ("error out"=w104:errorcluster, "Plot Names Notifier Ref"=w103:refnum<notifier>)  [unwired: 1 in, 9 out]
            n165 = Send Notification(notification=w102, notifier=w103, error in (no error)=w104) -> ()  [unwired: 2 out]
          }
        }
        n166 = case shown="Default" w97 {
          tunnel: w96 -> [w109 _]
          frame Default {
            n167 = call <vilib>:"Temp Scene Update.vi"("Property Name"=Temp_Scene_Property_Action."Plot Specific Property", "State"=Temp_Scene_State."Update Scene", "Property In"=w109) -> ()  [unwired: 3 in, 6 out]
          }
          frame "Exit" {
          }
        }
      }
      frame "Exit" {
      }
    }
  }
  "Mesh Property Out" <- w15
